vi "Actor test.vi"(0 "Class Actor Test IN":refnum<class "Actor Test (Default).lvclass">, 11 "entrée d'erreur (pas d'erreur)":errorcluster) -> (4 "Class Actor Test Out":refnum<class "Actor Test (Default).lvclass">, 6 "Results":bool[](array[boolean]), 8 "Tableau":T3(array[cluster]), 10 "Stopped":bool, 15 "sortie d'erreur":errorcluster)   [LabVIEW 2020, in "Library Core.lvlib" / "Actor Test (Default).lvclass"]
uses:
  Actor Test (Default).lvclass
  Commun VI/TypeDef/Commande Test/Commande Value Type.ctl
  Commun VI/TypeDef/Commande Test/Commande Type Test.ctl
  Software/Standard TB/Function/Type DEF/Commande Gestion Execution Scenario.ctl
  Sequencer (Default)/Sequencer (Default).lvclass
  Instrument/Instrument (Default)/Class Instrument (Default).lvclass
  Test/Test (Default)/Test (Default).lvclass
  Actor Test (Default).lvclass/Actor Test (Default).ctl
  Commun VI/Library Commun.lvlib
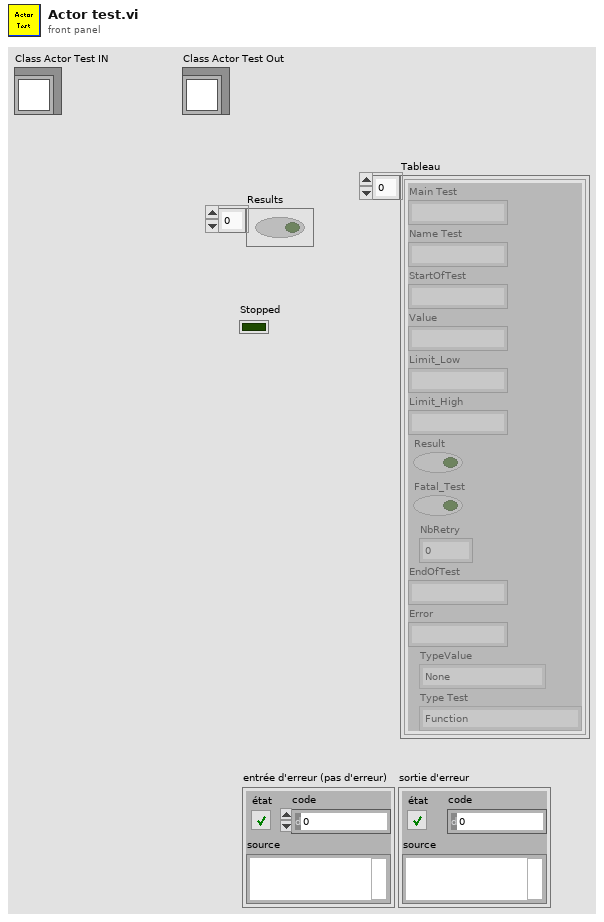
[diagram p1: front panel]
types:
  T1 = typedef "Library Commun.lvlib/Commande Value Type.ctl" = enum16{"None", "String", "Number", "Timestamp", "Boolean", "Array"}
  T2 = typedef "Library Commun.lvlib/Commande Type Test.ctl" = enum16{"Function", "Test", "Calculation"}
  T3 = cluster{"Main Test":string, "Name Test":string, "StartOfTest":string, "Value":string, "Limit_Low":string, "Limit_High":string, "Result":bool, "Fatal_Test":bool, "NbRetry":dbl, "EndOfTest":string, "Error":string, "TypeValue":T1, "Type Test":T2}[]
  T4 = typedef "Commande Gestion Execution Scenario.ctl" = cluster{"Name Test":string, "Etat":cluster{"Menu déroulant":u16}, "Affiche result":bool, "Tab Test Result":cluster{"Main Test":string, "Name Test":string, "StartOfTest":string, "Value":string, "Limit_Low":string, "Limit_High":string, "Result":bool, "Fatal_Test":bool, "NbRetry":dbl, "EndOfTest":string, "Error":string, "TypeValue":T1, "Type Test":T2}[], "State Test":string}
  T5 = cluster{"Type Function":string, "Test Name":string, "Class launched by the actors ":string, "Name_Instrument":string, "Class_Instrument":string, "Parameter (Json)":string, "Limit_Low":string, "Limit_Hight":string, "Fatal Test ?":bool, "Parallelized ?":bool, "Mandatory ?":bool}[]
  T6 = cluster{"Event Error":refnum<user-event>, "Data test ":refnum<user-event>, "Stop":refnum<user-event>, "Action in progress":refnum<user-event>, "Operator Shutdown":refnum<user-event>}
  T7 = enum16{"Get Loop Sequence", "Reset", "Set Loop Sequence"}
  T8 = enum16{"Get Test Class", "Set Test object", "Get Test object", "List Test", "Init"}
  T9 = enum16{"Add Instr", "Remove Instr", "List Instr", "Get Instr Class", "Get Instr obj", "Save Insrt obj", "Modify Insrt obj", "Init"}
  T10 = typedef "Library Commun.lvlib/Commande Data Test.ctl" = cluster{"Main Test":string, "Name Test":string, "StartOfTest":string, "Value":string, "Limit_Low":string, "Limit_High":string, "Result":bool, "Fatal_Test":bool, "NbRetry":dbl, "EndOfTest":string, "Error":string, "TypeValue":T1, "Type Test":T2}
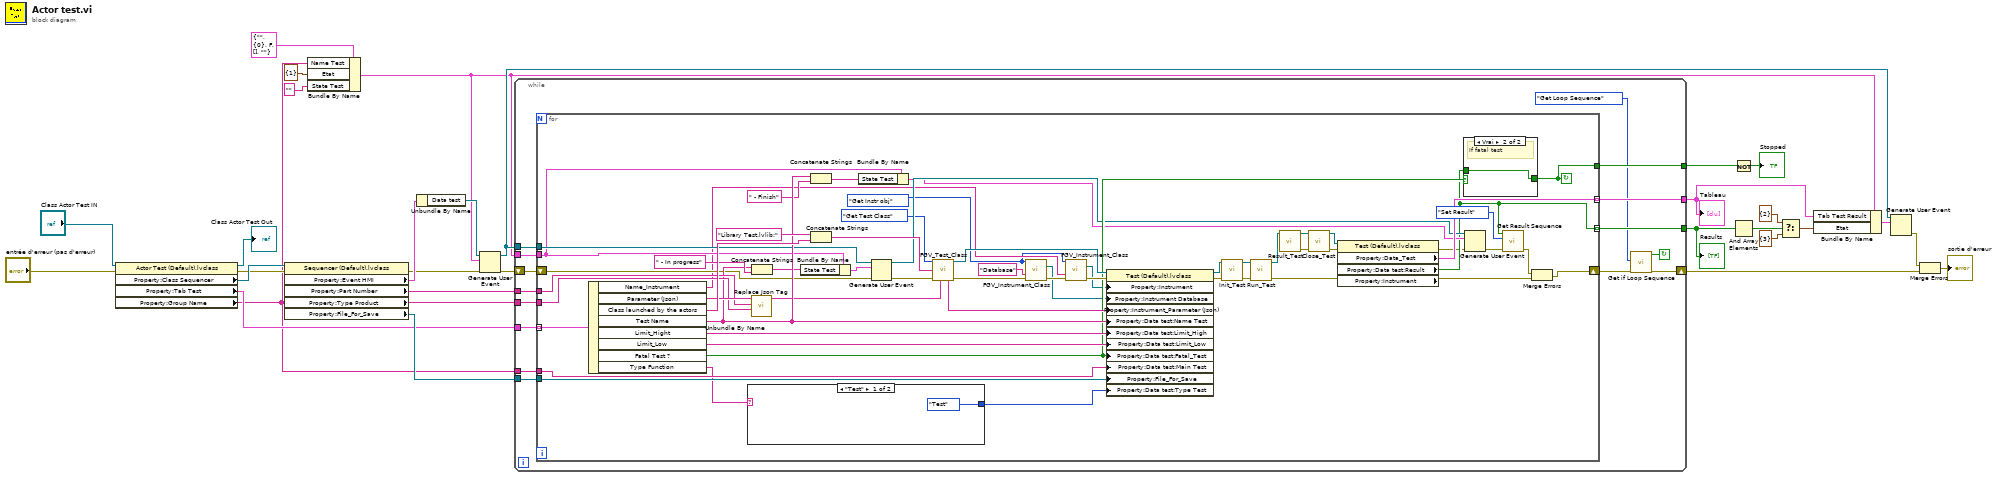
[diagram p0: block diagram]
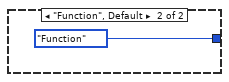
[diagram p2: hidden frame]
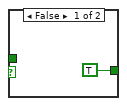
[diagram p3: hidden frame]
diagram:
  n1 = property class="Actor Test (Default).lvclass"(reference="Class Actor Test IN", error in="entrée d'erreur (pas d'erreur)") -> (reference out=→"Class Actor Test Out":refnum<class "Actor Test (Default).lvclass">, error out=w13:errorcluster, "Property:Class Sequencer"=w15:refnum<class "Sequencer (Default).lvclass">, "Property:Tab Test"=w16:T5, "Property:Group Name"=w5:string)
  n2 = property class="Sequencer (Default).lvclass"(reference=w15, error in=w13) -> (error out=w18:errorcluster, "Property:Event HMI"=w28:T6, "Property:Part Number"=w31:string, "Property:Type Product"=w30:string, "Property:File_For_Save"=w29:refnum<queue>)  [unwired: 1 out]
  n3 = Bundle By Name(cluster=T4 {"Name Test"="", "Etat"={"Menu déroulant"=0}, "Affiche result"=FALSE, "Tab Test Result"=[], "State Test"=""} ("élément"), "Name Test"=w5, "Etat"=cluster{"Menu déroulant":u16} {"Menu déroulant"=1}, "State Test"="") -> (w7:T4)
  n4 = Unbundle By Name(w28) -> ("Data test"=w19:refnum<user-event>)
  n5 = Generate User Event(user event=w19, event data cluster=w7, error in=w18) -> (user event out=w9:refnum<user-event>, error out=w1:errorcluster)  [unwired: 1 in]
  n6 = while {
    tunnel: w31 -> [w46]
    tunnel: w30 -> [w45]
    tunnel: w29 -> [w44]
    tunnel: [w43] -> w22
    tunnel: w16 -> [w42]
    tunnel: [w41] -> w11
    tunnel: w9 -> [w40]
    tunnel: w7 -> [w39]
    tunnel: w5 -> [w38]
    tunnel: [w37] -> w2
    shift-right: [w34] -> w3
    shift-left: w1 -> [w36]
    stop <- w33 continue-if-true
    n7 = for {
      tunnel: [w88] -> w37 mode=indexing
      tunnel: w42 -> [w89] mode=indexing
      shift-right: [w47] -> w35
      shift-left: w36 -> [w78]
      tunnel: [w61] -> w43 mode=indexing
      tunnel: w45 -> [w95]
      tunnel: w46 -> [w94]
      tunnel: w44 -> [w91]
      tunnel: w38 -> [w90]
      tunnel: [w79] -> w41
      tunnel: w40 -> [w77]
      tunnel: w39 -> [w72]
      stop <- w79 continue-if-true
      w48 = T9."Get Instr obj" ("Action")
      n8 = Unbundle By Name(w89) -> ("Name_Instrument"=w49:string, "Parameter (Json)"=w96:string, "Class launched by the actors"=w99:string, "Test Name"=w86:string, "Limit_Hight"=w93:string, "Limit_Low"=w92:string, "Fatal Test ?"=w80:bool, "Type Function"=w60:string)
      n9 = case shown="\"Test\"" w60 {
        tunnel: [Commande_Type_Test."Test" ("Type Test") Commande_Type_Test."Function" ("Type Test")] -> w59
        frame "Test" {
        }
        frame "Function", Default {
        }
      }
      n10 = call "Replace Json Tag.vi"("Part Number PCBA"=w95, "Type Product"=w94, "Parameter (Json) en entrée"=w96) -> ("Parameter (Json) en sortie"=w82:string)  [unwired: 8 in]
      n11 = Concatenate Strings(w86, " - In progress" ("chaîne")) -> (w75:string)
      n12 = Bundle By Name(cluster=w72, "State Test"=w75) -> (w76:T4)
      n13 = Concatenate Strings(w86, " - Finish" ("chaîne")) -> (w71:string)
      n14 = Concatenate Strings("Library Test.lvlib:", w99) -> (w84:string)
      n15 = Bundle By Name(cluster=w72, "State Test"=w71) -> (w70:T4)
      n16 = Generate User Event(user event=w77, event data cluster=w76, error in=w78) -> (user event out=w73:refnum<user-event>, error out=w74:errorcluster)  [unwired: 1 in]
      n17 = call "FGV_Test_Class.vi"("Action"=T8."Get Test Class", "Test class"=w84, "error in (no error)"=w74, "Parameter (Json) en entrée"=w82) -> ("Test (Default).lvclass"=w83:refnum<class "Test (Default).lvclass">, "Parameter (Json) en sortie"=w81:string, "error out"=w67:errorcluster)  [unwired: 8 in, 1 out]
      n18 = call "FGV_Instrument_Class.vi"("Action"=w48, "Instr name"="Database", "error in (no error)"=w67) -> ("Familly class Out"=w65:refnum<class "Class Instrument (Default).lvclass">, "error out"=w66:errorcluster)  [unwired: 10 in, 1 out]
      n19 = call "FGV_Instrument_Class.vi"("Action"=w48, "Instr name"=w49, "error in (no error)"=w66) -> ("Familly class Out"=w58:refnum<class "Class Instrument (Default).lvclass">, "error out"=w101:errorcluster)  [unwired: 10 in, 1 out]
      n20 = property class="Test (Default).lvclass"(reference=w83, error in=w101, "Property:Instrument"=w58, "Property:Instrument Database"=w65, "Property:Instrument_Parameter (Json)"=w81, "Property:Data test:Name Test"=w86, "Property:Data test:Limit_High"=w93, "Property:Data test:Limit_Low"=w92, "Property:Data test:Fatal_Test"=w80, "Property:Data test:Main Test"=w90, "Property:File_For_Save"=w91, "Property:Data test:Type Test"=w59) -> (reference out=w97:refnum<class "Test (Default).lvclass">, error out=w98:errorcluster)
      n21 = call-dynamic "Init_Test.vi"("error in (no error)"=w98, "Test (Default) en entrée"=w97) -> ("error out"=w68:errorcluster, "Test (Default) en sortie"=w102:refnum<class "Test (Default).lvclass">)  [unwired: 8 in]
      n22 = call-dynamic "Run_Test.vi"("error in (no error)"=w68, "Test (Default) en entrée"=w102) -> ("error out"=w50:errorcluster, "Test (Default) en sortie"=w57:refnum<class "Test (Default).lvclass">)  [unwired: 8 in]
      n23 = call-dynamic "Result_Test.vi"("Test (Default) en entrée"=w57) -> ("error out"=w55:errorcluster, "Test (Default) en sortie"=w54:refnum<class "Test (Default).lvclass">)  [unwired: 9 in]
      n24 = call-dynamic "Close_Test.vi"("error in (no error)"=w55, "Test (Default) en entrée"=w54) -> ("error out"=w52:errorcluster, "Test (Default) en sortie"=w53:refnum<class "Test (Default).lvclass">)  [unwired: 8 in]
      n25 = property class="Test (Default).lvclass" props=["Property:Data_Test", "Property:Data test:Result", "Property:Instrument"](reference=w53, error in=w52) -> (error out=w56:errorcluster, "Property:Data_Test"=w88:T10, "Property:Data test:Result"=w61:bool)  [unwired: 2 out]
      n26 = case shown="Vrai" w80 {
        tunnel: w61 -> [_ w106]
        tunnel: [TRUE w106] -> w79
        frame False {
        }
        frame True {
          # "If fatal test"
        }
      }
      n27 = Generate User Event(user event=w73, event data cluster=w70, error in=w56) -> (error out=w63:errorcluster)  [unwired: 1 in, 1 out]
      n28 = call "Get Result Sequence.vi"("error in (no error)"=w63, "Function"=enum16{"Get Result", "Reset", "Set Result"}."Set Result", "Result In"=w61) -> ("error out"=w51:errorcluster)  [unwired: 7 in, 1 out]
      n29 = Merge Errors(w51, w50) -> (w47:errorcluster)
    }
    n30 = call "Get if Loop Sequence.vi"("error in (no error)"=w35, "Function"=T7."Get Loop Sequence") -> ("error out"=w34:errorcluster, "Loop Out"=w33:bool)  [unwired: 8 in]
  }
  "Tableau" <- w2
  "Results" <- w22
  n31 = Not(x=w11) -> (.not. x?=→"Stopped":bool)
  n32 = And Array Elements(Boolean array=w22) -> (logical AND=w26:bool)
  n33 = Select(t=cluster{"Menu déroulant":u16} {"Menu déroulant"=2} ("Etat"), s=w26, f=cluster{"Menu déroulant":u16} {"Menu déroulant"=3} ("Etat")) -> (s? t:f=w24:cluster{"Menu déroulant":u16})
  n34 = Bundle By Name(cluster=w7, "Tab Test Result"=w2, "Etat"=w24) -> (w27:T4)
  n35 = Generate User Event(user event=w9, event data cluster=w27) -> (error out=w21:errorcluster)  [unwired: 2 in, 1 out]
  n36 = Merge Errors(w21, w3) -> (→"sortie d'erreur":errorcluster)
